vi "Create.vi"(7 "VolatusAPI":refnum<class "VolatusAPI.lvclass">, 8 "error in (no error)":errorcluster, 9 "JSON":string, 10 "Ref":refnum<vi>, 11 "GUI Element in":refnum<class "GUI Element.lvclass">) -> (0 "error out":errorcluster, 3 "GUI Element out":refnum<class "GUI Element.lvclass">)   [LabVIEW 2020, in "VolatusGUI.lvlib" / "GUI Element.lvclass"]
uses:
  GUI Element.lvclass
  Volatus/VolatusAPI/VolatusAPI.lvclass
  GUI Element.lvclass/GUI Element.ctl
  f2390cbb-3f59-4de1-83a9-eb11a445dceb.vi
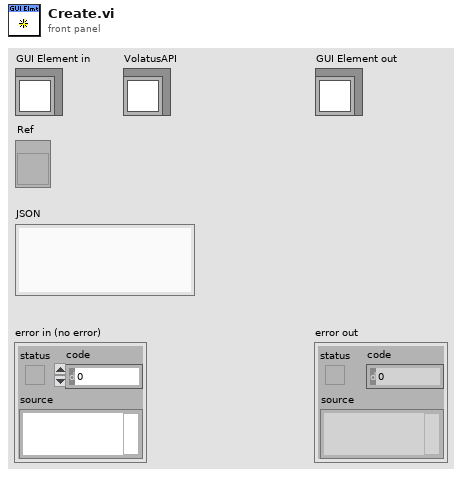
[diagram p1: front panel]
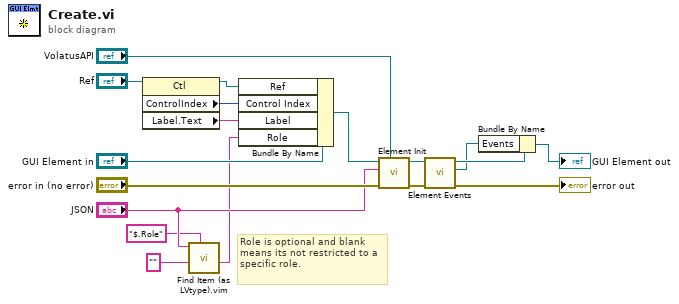
[diagram p0: block diagram]
diagram:
  # "Role is optional and blank means its not restricted to a specific role."
  n1 = property class="Ctl"(reference="Ref") -> (reference out=w12:refnum<vi>, "ControlIndex"=w11:i32, "Label.Text"=w5:string)  [unwired: 1 in, 1 out]
  n2 = call "Find Item (as LVtype).vim"("$Path or Item Name"="$.Role", "Data Type and Default Value"="", "JSON"="JSON") -> ("Data"=w1:string)  [unwired: 5 in, 3 out]
  n3 = Bundle By Name(cluster="GUI Element in", "Ref"=w12, "Control Index"=w11, "Label"=w5, "Role"=w1) -> (w14:refnum<class "GUI Element.lvclass">)
  n4 = call-dynamic "Element Init.vi"("VolatusAPI"="VolatusAPI", "error in (no error)"="error in (no error)", "JSON"="JSON", "GUI Element in"=w14) -> ("error out"=w15:errorcluster, "GUI Element out"=w9:refnum<class "GUI Element.lvclass">)  [unwired: 6 in]
  n5 = call-dynamic "Element Events.vi"("error in (no error)"=w15, "GUI Element in"=w9) -> ("error out"=→"error out":errorcluster, "Element Events"=w6:refnum<class "Control Event Registrations.lvclass">, "GUI Element out"=w8:refnum<class "GUI Element.lvclass">)  [unwired: 7 in]
  n6 = Bundle By Name(cluster=w8, "Events"=w6) -> (→"GUI Element out":refnum<class "GUI Element.lvclass">)
